vi "Create_File_Directories.vi"(8 "error in (no error)":errorcluster) -> (0 "error out":errorcluster)   [LabVIEW 2024]
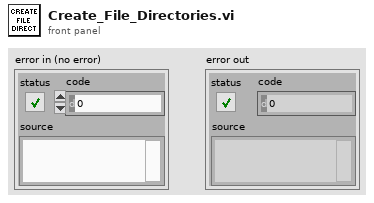
[diagram p1: front panel]
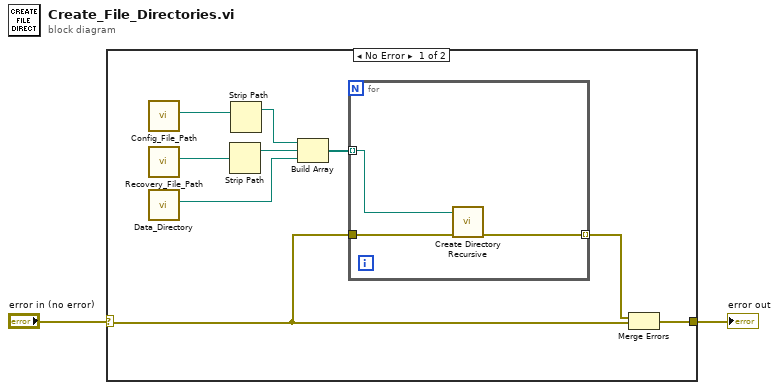
[diagram p0: block diagram]
diagram:
  n1 = case shown="No Error" "error in (no error)" {
    selector: "error in (no error)" -> [w9 w15]
    tunnel: [w10 w15] -> w1
    frame No Error {
      n2 = call "Config_File_Path.vi"() -> ("Config File Path"=w6:path)  [unwired: 11 in]
      n3 = call "Recovery_File_Path.vi"() -> ("Recovery File Path"=w4:path)  [unwired: 11 in]
      n4 = call "Data_Directory.vi"() -> ("Data Directory"=w11:path)  [unwired: 11 in]
      n5 = Strip Path(path=w4) -> (stripped path=w3:path)  [unwired: 1 out]
      n6 = Strip Path(path=w6) -> (stripped path=w5:path)  [unwired: 1 out]
      n7 = Build Array(w5, w3, w11) -> (w7:path[])
      n8 = for {
        tunnel: [w13] -> w8 mode=indexing
        tunnel: w9 -> [w14]
        tunnel: w7 -> [w12] mode=indexing
        n9 = call <vilib>:"Create Directory Recursive.vi"("error in (no error)"=w14, "directory"=w12) -> ("error out"=w13:errorcluster)  [unwired: 3 in, 2 out]
      }
      n10 = Merge Errors(w8, w9) -> (w10:errorcluster)
    }
    frame Error {
    }
  }
  "error out" <- w1
